vi "Action_Template.vi"(0 "Sequence Context In":refnum<k7>, 5 "error in (no error)":errorcluster) -> (14 "Sequence Context Out":refnum<k7>, 19 "error out":errorcluster)   [LabVIEW 2014]
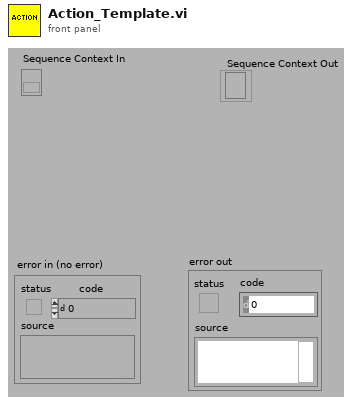
[diagram p1: front panel]
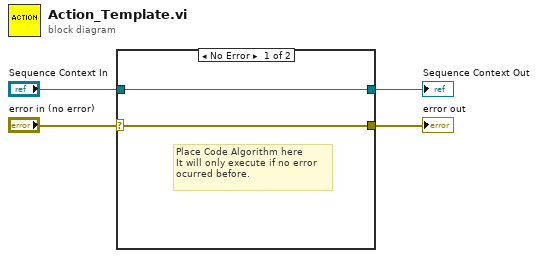
[diagram p0: block diagram]
diagram:
  n1 = case shown="No Error" "error in (no error)" {
    selector: "error in (no error)" -> [w6 w8]
    tunnel: "Sequence Context In" -> [w5 w7]
    tunnel: [w6 w8] -> w2
    tunnel: [w5 w7] -> w1
    frame No Error {
      # "Place Code Algorithm here\nIt will only execute if no error \nocurred before."
    }
    frame Error {
    }
  }
  "error out" <- w2
  "Sequence Context Out" <- w1
